vi "2D cross product.vi"(1 "B":dbl[](array[numeric])=[0.0, 0.0], 2 "A":dbl[](array[numeric])=[0.0, 0.0]) -> (0 "A X B":dbl)   [LabVIEW 2014]
panel:
  # "PN 30/08/2014"
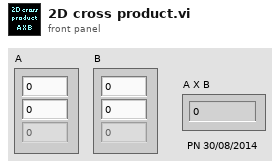
[diagram p1: front panel]
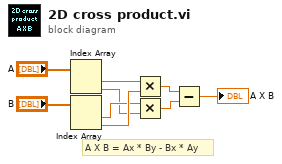
[diagram p0: block diagram]
diagram:
  # "A X B = Ax * By - Bx * Ay"
  n1 = Index Array(array="A") -> (element #1=w4:dbl, element #2=w1:dbl)  [unwired: 2 in]
  n2 = Index Array(array="B") -> (element #1=w2:dbl, element #2=w3:dbl)  [unwired: 2 in]
  n3 = Multiply(x=w4, y=w3) -> (x*y=w6:dbl)
  n4 = Multiply(x=w2, y=w1) -> (x*y=w7:dbl)
  n5 = Subtract(x=w6, y=w7) -> (x-y=→"A X B":dbl)
